vi "Label Visibility.vi"(6 "Show Text":bool, 8 "error in":errorcluster, 10 "Lithography Data":T2(array[cluster]), 11 "BigMAQ in":refnum<class "BigMAQ.lvclass">) -> (0 "error out":errorcluster, 3 "BigMAQ out":refnum<class "BigMAQ.lvclass">)   [LabVIEW 2019, in "BigMAQ.lvclass"]
uses:
  BigMAQ.lvclass
  <userlib>/LevyLab/Relay Box/Typedefs/Resistor--enum.ctl
  Overlay.ctl
  BigMAQ.lvclass/BigMAQ.ctl
  <userlib>/LevyLab/Relay Box/Relay-Box.lvclass
panel:
  out "Array":string[](array[string])
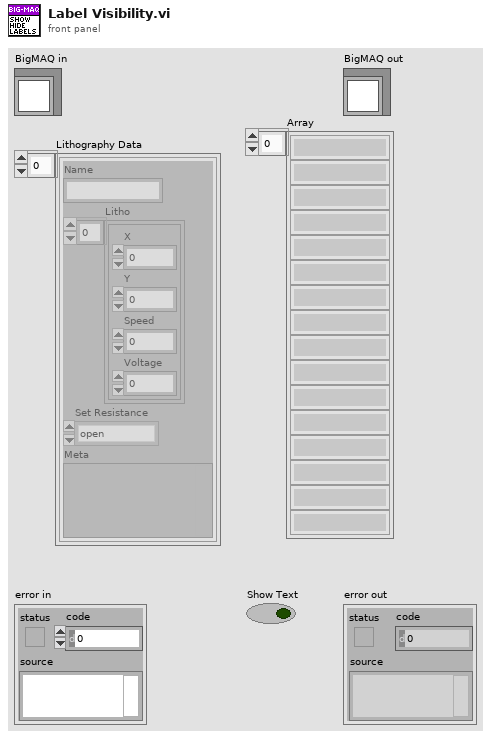
[diagram p1: front panel]
types:
  T1 = typedef "Relay-Box.lvclass/Resistor--enum.ctl" = enum16{"open", "discharge tip", "0 ohms", "100k ohm", "10M ohm", "1G ohm"}
  T2 = cluster{"Name":string, "Litho":cluster{"X":dbl, "Y":dbl, "Speed":dbl, "Voltage":dbl}[], "Set Resistance":T1, "Meta":variant}[]
  T3 = typedef "BigMAQ.lvclass/Overlay.ctl" = cluster{"Name":string, "Data":cluster{"Points":cluster{"X":dbl, "Y":dbl}[], "Voltages":dbl[]}}
  T4 = cluster{"X":dbl, "Y":dbl, "Speed":dbl, "Voltage":dbl}[]
  T5 = typedef "IMAQ Image.ctl" = refnum<image>
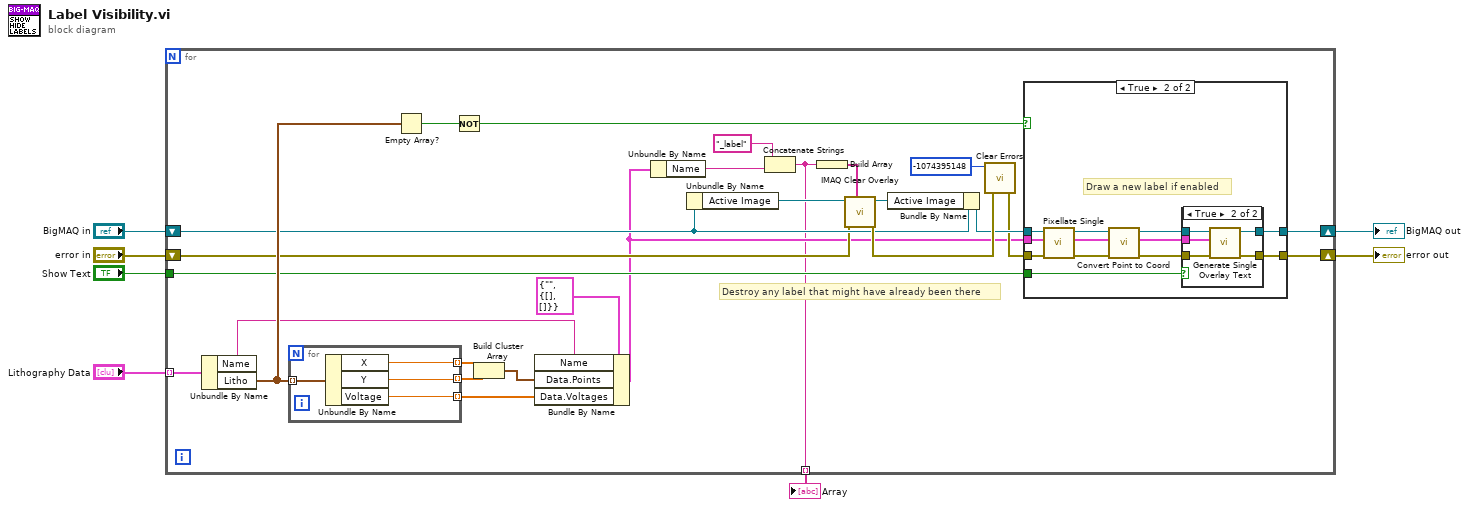
[diagram p0: block diagram]
diagram:
  n1 = for {
    tunnel: "Lithography Data" -> [w25] mode=indexing
    tunnel: "Show Text" -> [w23]
    shift-right: [w21] -> w5
    shift-left: "error in" -> [w11]
    shift-right: [w22] -> w6
    shift-left: "BigMAQ in" -> [w14]
    tunnel: [w8] -> w1 mode=indexing
    # "Destroy any label that might have already been there"
    n2 = Unbundle By Name(w25) -> ("Name"=w29:string, "Litho"=w31:T4)
    n3 = for {
      tunnel: w31 -> [w55] mode=indexing
      tunnel: [w58] -> w30 mode=indexing
      tunnel: [w57] -> w27 mode=indexing
      tunnel: [w56] -> w28 mode=indexing
      n4 = Unbundle By Name(w55) -> ("X"=w57:dbl, "Y"=w56:dbl, "Voltage"=w58:dbl)
    }
    n5 = Empty Array?(array=w31) -> (empty?=w32:bool)
    n6 = Not(x=w32) -> (.not. x?=w24:bool)
    n7 = Build Cluster Array(w27, w28) -> (w26:cluster{"X":dbl, "Y":dbl}[])
    n8 = Bundle By Name(cluster=T3 {"Name"="", "Data"={"Points"=[], "Voltages"=[]}} ("Overlay"), "Name"=w29, "Data.Points"=w26, "Data.Voltages"=w30) -> (w10:T3)
    n9 = Unbundle By Name(w10) -> ("Name"=w9:string)
    n10 = Unbundle By Name(w14) -> ("Active Image"=w15:T5)
    n11 = Concatenate Strings("_label" ("string"), w9) -> (w8:string)
    n12 = Build Array(w8) -> (w19:string[])
    n13 = call "IMAQ Clear Overlay"("Groups"=w19, "error in (no error)"=w11, "Image"=w15) -> ("error out"=w17:errorcluster, "Image Out"=w16:T5)  [unwired: 7 in]
    n14 = Bundle By Name(cluster=w14, "Active Image"=w16) -> (w13:refnum<class "BigMAQ.lvclass">)
    n15 = call <vilib>:"Clear Errors.vi"("error in (no error)"=w17, "specific error code to clear (0: all)"=-1074395148) -> ("error out"=w12:errorcluster)  [unwired: 4 in, 1 out]
    n16 = case shown="True" w24 {
      tunnel: w10 -> [_ w47]
      tunnel: [w35 w43] -> w21
      tunnel: [w34 w42] -> w22
      tunnel: w23 -> [_ w41]
      tunnel: w12 -> [w35 w40]
      tunnel: w13 -> [w34 w39]
      frame False {
        # "Dont do anything for disabled objects"
      }
      frame True {
        # "Draw a new label if enabled"
        n17 = call "Pixellate Single.vi"("error in"=w40, "Overlay"=w47, "BigMAQ in"=w39) -> ("error out"=w44:errorcluster, "Pixellated Overlay"=w46:T3, "BigMAQ out"=w45:refnum<class "BigMAQ.lvclass">)  [unwired: 6 in]
        n18 = call "Convert Point to Coord.vi"("error in"=w44, "Overlay"=w46, "BigMAQ in"=w45) -> ("error out"=w38:errorcluster, "output cluster"=w36:T3, "BigMAQ out"=w37:refnum<class "BigMAQ.lvclass">)  [unwired: 5 in, 1 out]
        n19 = case shown="True" w41 {
          tunnel: w36 -> [_ w54]
          tunnel: w37 -> [w49 w53]
          tunnel: w38 -> [w48 w52]
          tunnel: [w48 w51] -> w43
          tunnel: [w49 w50] -> w42
          frame False {
          }
          frame True {
            n20 = call "Generate Single Overlay Text.vi"("error in"=w52, "Overlay"=w54, "BigMAQ in"=w53) -> ("error out"=w51:errorcluster, "BigMAQ out"=w50:refnum<class "BigMAQ.lvclass">)  [unwired: 7 in]
          }
        }
      }
    }
  }
  "error out" <- w5
  "BigMAQ out" <- w6
  "Array" <- w1
